vi "select bl section.vi"(1 "error in (no error)":errorcluster, 2 "Beamline selection":T1, 3 "reference":refnum<vi>) -> (0 "error out":errorcluster)   [LabVIEW 2016, in "main.lvlib"]
doc: "select bl section.vi takes the user's \"Beamline Section\" selection, transforms the enum\nrelated to the selection into a VI ref in the sub-VI case select bl section.vi, \nand inserts it into the lower sub-panel."
uses:
  main.lvlib
  beamline selection.ctl
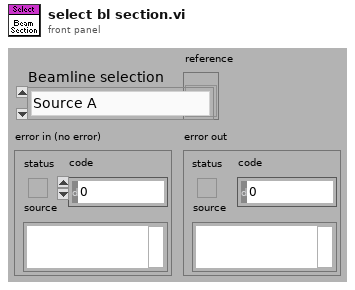
[diagram p1: front panel]
types:
  T1 = typedef "main.lvlib/beamline selection.ctl" = enum16{"Source A", "Source B", "Low Energy End", "High Energy End", "Transmission", "R30", "R45"}
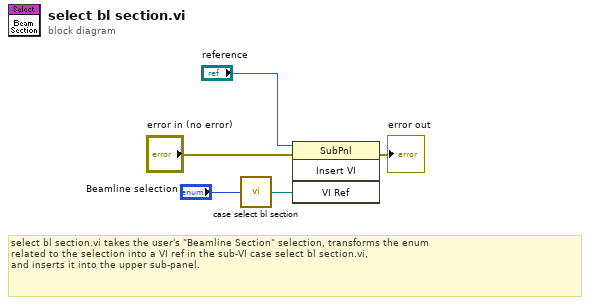
[diagram p0: block diagram]
diagram:
  # "select bl section.vi takes the user's \"Beamline Section\" selection, transforms the enum\nrelated to the selection into a VI ref in the sub-VI case select bl section.vi, \nand inserts it into the upper sub-panel."
  n1 = call "case select bl section.vi"("Beamline Section"="Beamline selection") -> ("VI Refnum"=w2:refnum<vi>)
  n2 = invoke on="Invoke Node" class="SubPnl" method="Insert VI"(reference="reference", error in="error in (no error)", "VI Ref"=w2) -> (error out=→"error out":errorcluster)  [unwired: 1 in, 3 out]
